vi "000 Driver Message.vi"(8 "error in":errorcluster caption="Error In", 11 "Queue In":T1={"UI"=refnum, "Message"=refnum, "Data"=refnum, "Caller"=refnum, "Name"="000 Common", "Data Path"=path "", "Class Path"=path "", "SubPanel"=refnum, "Project Name"="", "MNT"="", "Title"="", "Data Source"=refnum, "Queue List"={}, "VI"=refnum, "UE"=refnum}) -> (0 "error out":errorcluster caption="Error Out", 2 "Queue NUmber":i32, 3 "Queue Out":T1={"UI"=refnum, "Message"=refnum, "Data"=refnum, "Caller"=refnum, "Name"="000 Common", "Data Path"=path "", "Class Path"=path "", "SubPanel"=refnum, "Project Name"="", "MNT"="", "Title"="", "Data Source"=refnum, "Queue List"={}, "VI"=refnum, "UE"=refnum})   [LabVIEW 2020]
uses:
  000 Module Data Type.ctl
  Queue Message.ctl
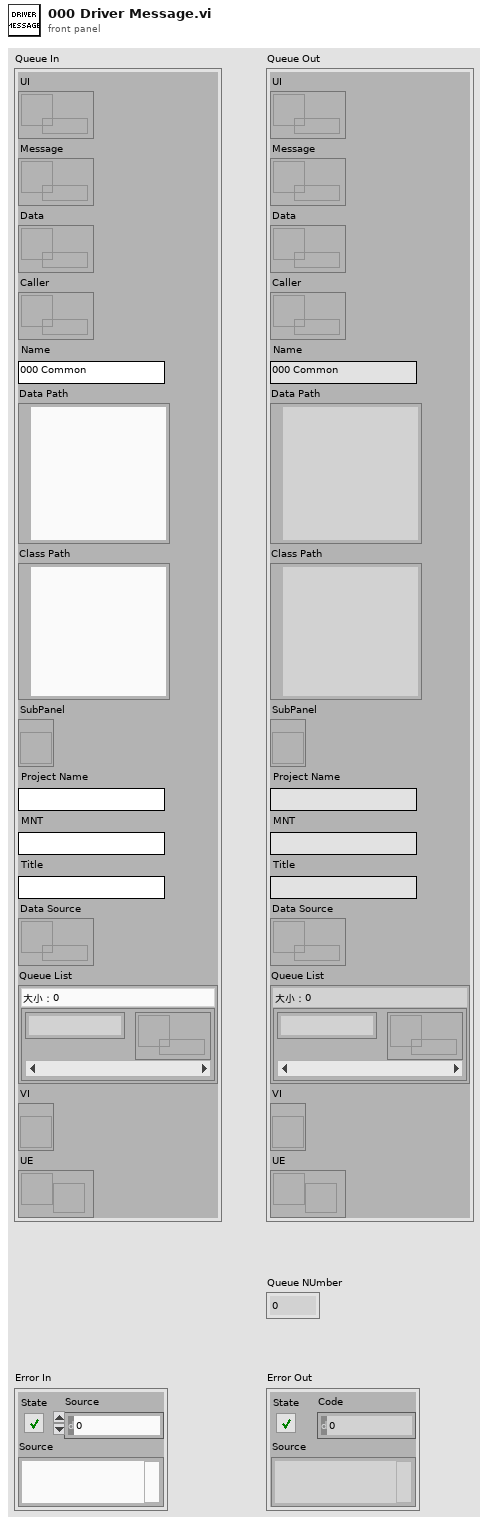
[diagram p1: front panel]
types:
  T1 = typedef "000 Module Data Type.ctl" = cluster{"UI":refnum<queue>, "Message":refnum<queue>, "Data":refnum<queue>, "Caller":refnum<queue>, "Name":string, "Data Path":path, "Class Path":path, "SubPanel":refnum<vi>, "Project Name":string, "MNT":string, "Title":string, "Data Source":refnum<queue>, "Queue List":map{string, refnum<queue>}, "VI":refnum<vi>, "UE":refnum<user-event>}
  T2 = enum32{"Invalid", "Standard", "Closed", "Hidden", "Minimized", "Maximized"}
  T3 = cluster{"Caller":refnum<queue>, "Message":refnum<queue>}
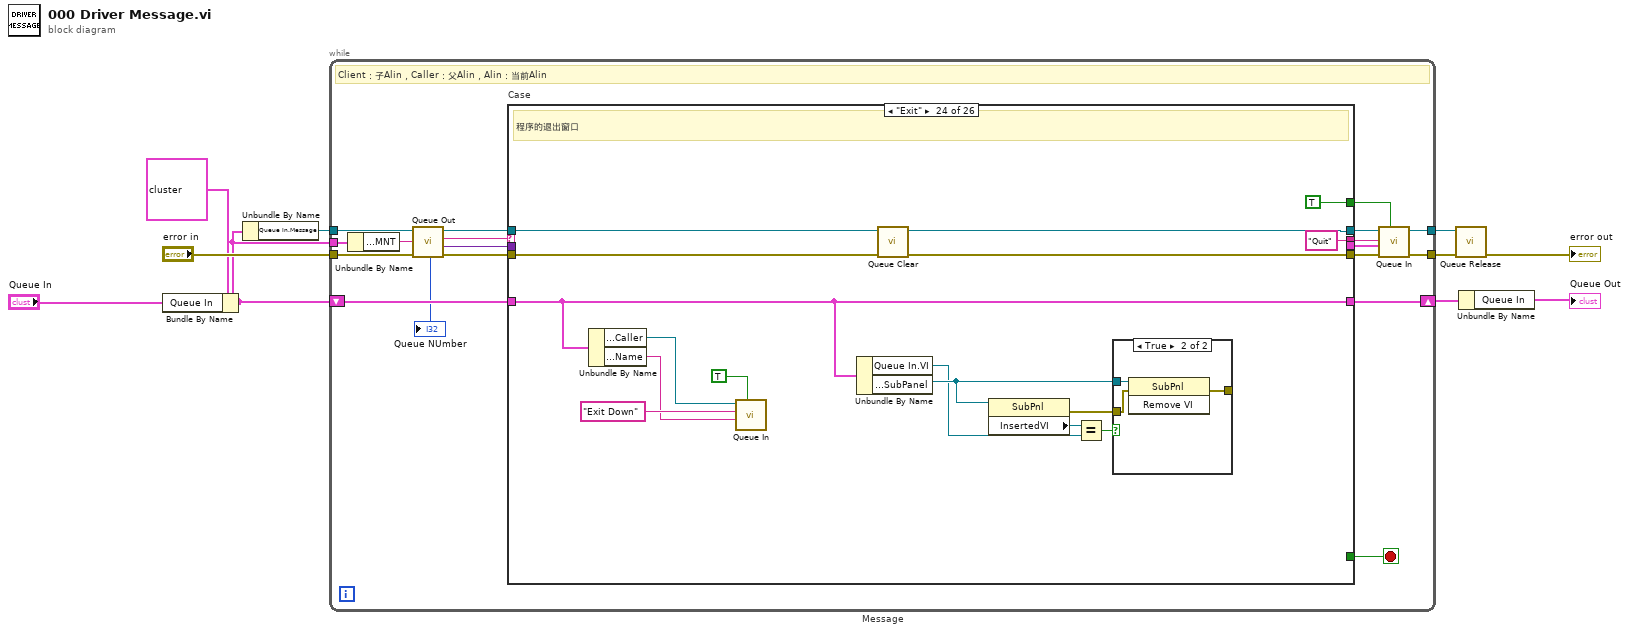
[diagram p0: block diagram]
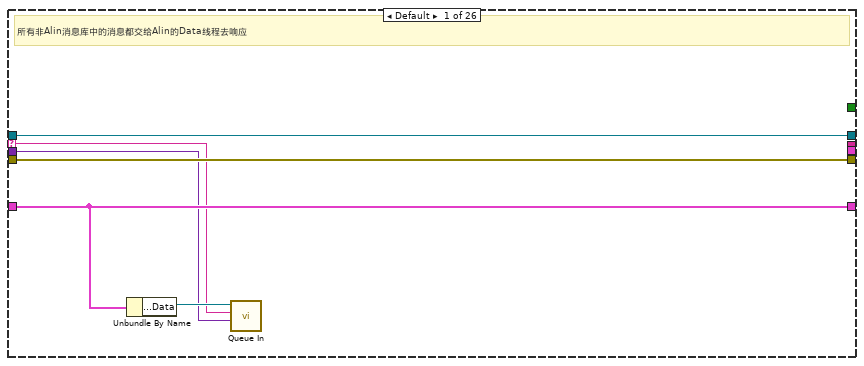
[diagram p2: hidden frame]
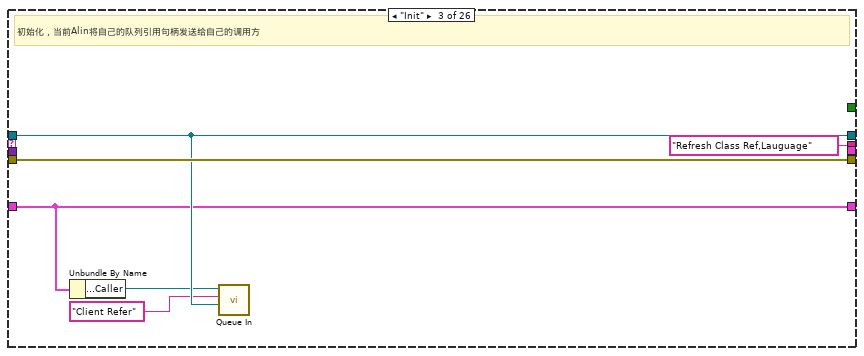
[diagram p4: hidden frame]
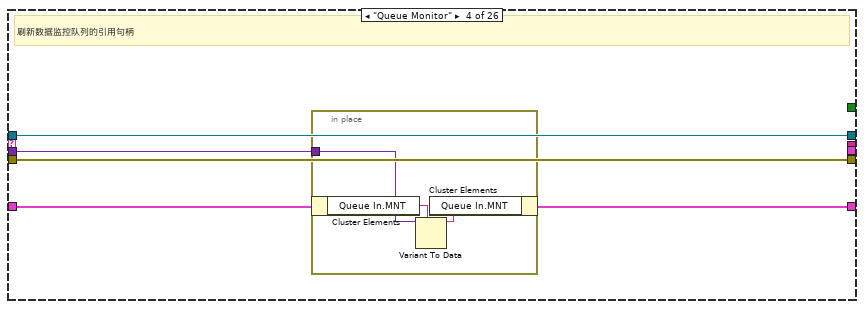
[diagram p5: hidden frame]
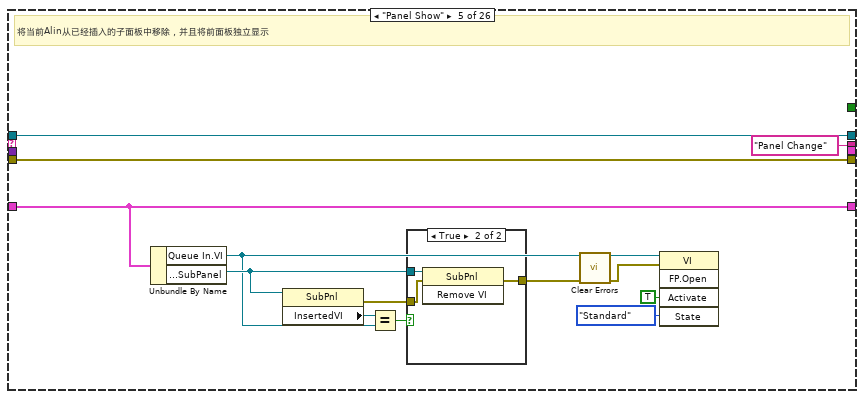
[diagram p6: hidden frame]
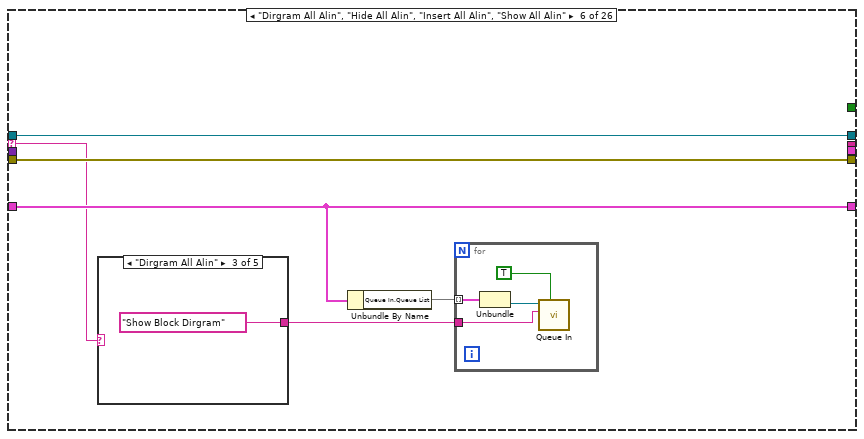
[diagram p8: hidden frame]
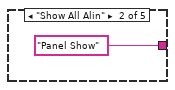
[diagram p10: hidden frame]
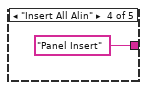
[diagram p11: hidden frame]
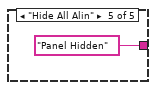
[diagram p12: hidden frame]
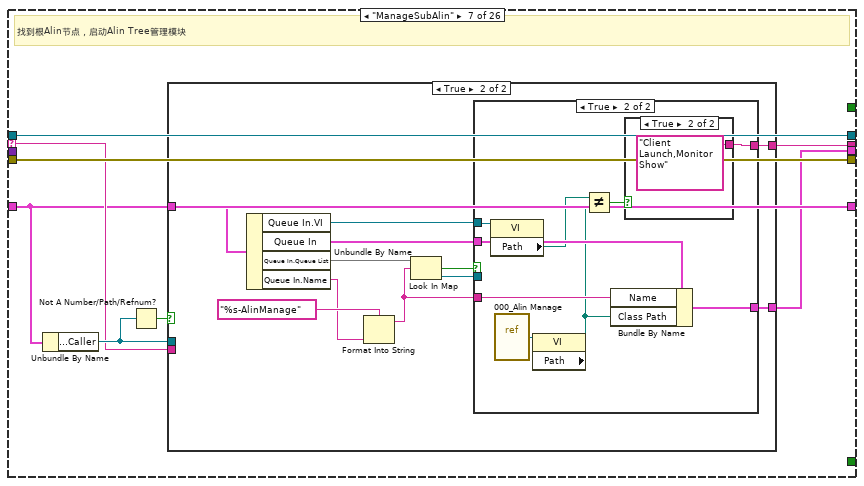
[diagram p13: hidden frame]
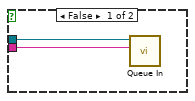
[diagram p14: hidden frame]
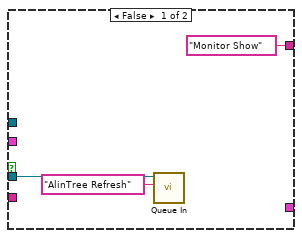
[diagram p15: hidden frame]
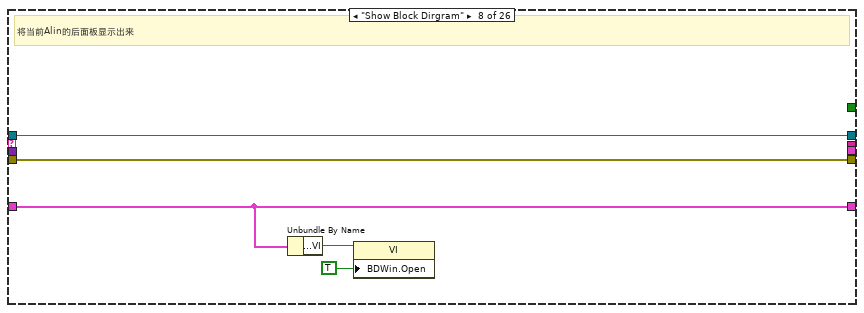
[diagram p17: hidden frame]
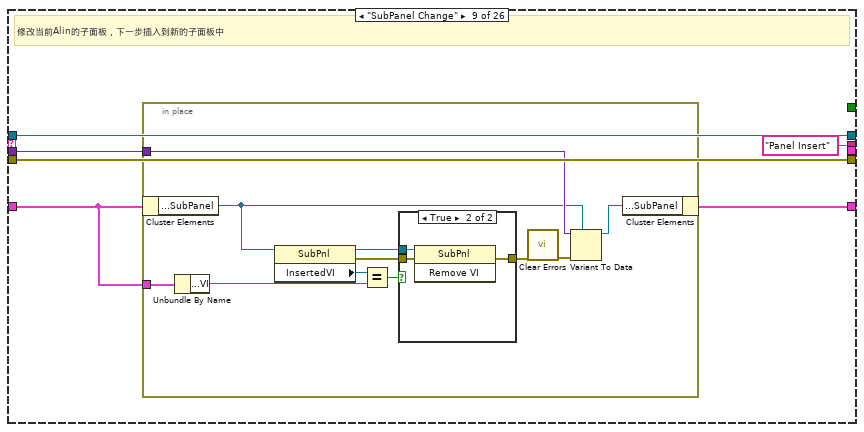
[diagram p18: hidden frame]
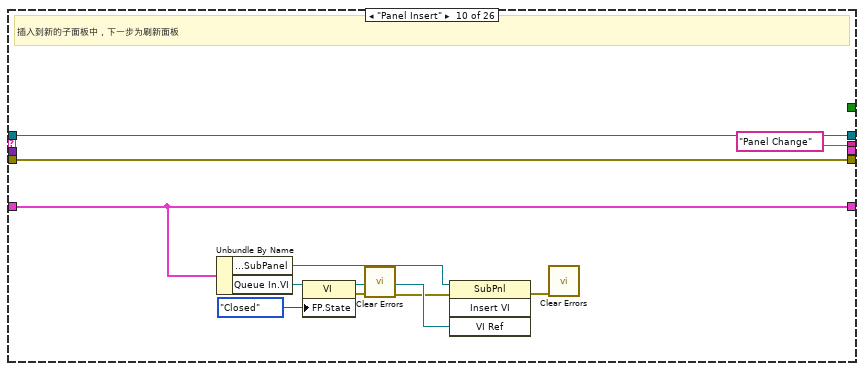
[diagram p20: hidden frame]
diagram:
  n1 = Bundle By Name ("按名称捆绑")(cluster=cluster{"Queue In":T1} {"Queue In"={"UI"=refnum, "Message"=refnum, "Data"=refnum, "Caller"=refnum, "Name"="000 Common", "Data Path"=path "", "Class Path"=path "", "SubPanel"=refnum, "Project Name"="", "MNT"="", "Title"="", "Data Source"=refnum, "Queue List"={}, "VI"=refnum, "UE"=refnum}}, "Queue In"="Queue In") -> (w3:cluster{"Queue In":T1})
  n2 = Unbundle By Name ("按名称解除捆绑")(w3) -> ("Queue In.Message"=w8:refnum<queue>)
  n3 = while "Message" {
    tunnel: w8 -> [w25]
    tunnel: [w22] -> w9
    tunnel: [w21] -> w10
    shift-right: [w18] -> w2
    shift-left: w3 -> [w17]
    tunnel: "error in" -> [w16]
    tunnel: w3 -> [w14]
    stop <- w29 stop-if-true
    # "Client：子Alin，Caller：父Alin，Alin：当前Alin"
    n4 = Unbundle By Name ("按名称解除捆绑")(w14) -> ("Queue In.MNT"=w13:string)
    n5 = call "Queue Out.vi"("error in (no error)"=w16, "Monitor"=w13, "Queue In"=w25) -> ("error out"=w28:errorcluster, "Data"=w26:variant, "Message"=w27:string, "Queue Out"=w24:refnum<queue>, "Queue NUmber"=→"Queue NUmber":i32)  [unwired: 4 in]
    n6 = case "Case" shown="\"Exit\"" w27 {
      selector: w27 -> [w31 _ _ _ _ w69 w86 _ _ _ _ w162 w173 _ _ w223 w235 w249 _ _ w278 _ _ _ _ _]
      tunnel: w24 -> [w35 w38 w43 w49 w65 w74 w90 w121 w127 w152 w158 w167 w176 w188 w205 w225 w237 w254 w265 w277 w287 w305 w324 w344 w351 w355]
      tunnel: w28 -> [w34 w37 w44 w48 w64 w73 w89 w120 w126 w151 w157 w166 w175 w191 w209 w224 w240 w253 w264 w276 w286 w304 w323 w342 w352 w354]
      tunnel: [w35 w38 w43 w49 w65 w74 w90 w121 w127 w152 w158 w167 w171 w188 w205 w225 w237 w254 w265 w277 w287 w305 w324 w343 w351 w355] -> w23
      tunnel: [w34 w37 w44 w48 w64 w73 w89 w120 w126 w151 w157 w166 w174 w191 w209 w224 w240 w253 w264 w276 w286 w304 w323 w341 w352 w354] -> w20
      tunnel: [_ _ "Refresh Class Ref,Lauguage" _ "Panel Change" _ w83 _ "Panel Insert" "Panel Change" _ _ _ "Send Client Refer" _ "Refresh Class Ref" "Refresh Class Ref" "" _ _ "Exit Check" w297 "Exit Check,Refresh Class Ref" "Quit" _ _] -> w19
      tunnel: [_ _ _ _ _ _ _ _ _ _ _ _ _ _ _ _ _ _ _ _ _ _ _ _ TRUE _] -> w29
      tunnel: w26 -> [w30 _ _ w45 _ _ _ _ w123 _ _ _ _ w189 w208 _ w236 _ _ w272 _ _ w320 _ _ _]
      tunnel: [w33 w36 w40 w46 w63 w72 w85 w119 w124 w150 w154 w165 w180 w190 w198 w222 w239 w248 w263 w275 w284 w303 w321 w330 w349 w353] -> w18
      tunnel: w17 -> [w33 w36 w40 w47 w63 w72 w85 w119 w122 w150 w154 w165 w180 w185 w198 w222 w239 w248 w263 w275 w284 w303 w322 w330 w349 w353]
      tunnel: [_ _ _ _ _ _ _ _ _ _ _ _ _ _ _ _ _ _ _ _ _ w296 _ TRUE _ _] -> w12
      tunnel: [_ _ _ _ _ _ w84 _ _ _ _ _ _ _ _ _ _ _ _ _ _ _ _ _ _ _] -> w11
      frame Default {
        # "所有非Alin消息库中的消息都交给Alin的Data线程去响应"
        n7 = Unbundle By Name(w33) -> ("Queue In.Data"=w32:refnum<queue>)
        n8 = call "Queue In.vi"("Data"=w30, "Message"=w31, "Queue In"=w32) -> ()  [unwired: 7 in, 2 out]
      }
      frame "====System Message Start===" {
      }
      frame "Init" {
        # "初始化，当前Alin将自己的队列引用句柄发送给自己的调用方"
        n9 = Unbundle By Name(w40) -> ("Queue In.Caller"=w41:refnum<queue>)
        n10 = call "Queue In.vi"("Data"=w43, "Message"="Client Refer", "Queue In"=w41) -> ()  [unwired: 7 in, 2 out]
      }
      frame "Queue Monitor" {
        # "刷新数据监控队列的引用句柄"
        n11 = in-place {
          in-place-border: w45 -> [w52]
          n12 = in-place-cluster #1(w47) -> ("Queue In.MNT"=w51:string)
          n13 = Variant To Data(type=w51, Variant=w52) -> (data=w50:string)  [unwired: 1 in, 1 out]
          n14 = in-place-cluster #1("Queue In.MNT"=w50) -> (w46:cluster{"Queue In":T1})
        }
      }
      frame "Panel Show" {
        # "将当前Alin从已经插入的子面板中移除，并且将前面板独立显示"
        n15 = Unbundle By Name(w63) -> ("Queue In.VI"=w55:refnum<vi>, "Queue In.SubPanel"=w57:refnum<vi>)
        n16 = property class="SubPnl"(reference=w57) -> (error out=w53:errorcluster, "InsertedVI"=w56:refnum<vi>)  [unwired: 1 in, 1 out]
        n17 = Equal?(x=w56, y=w55) -> (x = y?=w54:bool)
        n18 = case shown="True" w54 {
          tunnel: [_ w68] -> w62
          tunnel: w57 -> [_ w67]
          tunnel: w53 -> [_ w66]
          frame False {
          }
          frame True {
            n19 = invoke class="SubPnl" method="Remove VI"(reference=w67, error in=w66) -> (error out=w68:errorcluster)  [unwired: 1 in, 2 out]
          }
        }
        n20 = call <vilib>:"Clear Errors.vi"("error in (no error)"=w62) -> ("error out"=w59:errorcluster)  [unwired: 5 in, 1 out]
        n21 = invoke class="VI" method="FP.Open"(reference=w55, error in=w59, "Activate"=TRUE ("激活？"), "State"=T2."Standard" ("状态")) -> ()  [unwired: 1 in, 5 out]
      }
      frame "Dirgram All Alin", "Hide All Alin", "Insert All Alin", "Show All Alin" {
        n22 = case shown="\"Dirgram All Alin\"" w69 {
          tunnel: [_ "Panel Show" ("Message") "Show Block Dirgram" ("Message") "Panel Insert" ("Message") "Panel Hidden" ("Message")] -> w70
          frame Default {
          }
          frame "Show All Alin" {
          }
          frame "Dirgram All Alin" {
          }
          frame "Insert All Alin" {
          }
          frame "Hide All Alin" {
          }
        }
        n23 = Unbundle By Name(w72) -> ("Queue In.Queue List"=w71:map{string, refnum<queue>})
        n24 = for {
          tunnel: w71 -> [w82] mode=indexing
          tunnel: w70 -> [w80]
          n25 = Unbundle(w82) -> ("Client Refer"=w81:refnum<queue>)  [unwired: 1 out]
          n26 = call "Queue In.vi"("First"=TRUE, "Message"=w80, "Queue In"=w81) -> ()  [unwired: 7 in, 2 out]
        }
      }
      frame "ManageSubAlin" {
        # "找到根Alin节点，启动Alin Tree管理模块"
        n27 = Unbundle By Name(w85) -> ("Queue In.Caller"=w87:refnum<queue>)
        n28 = Not A Number/Path/Refnum?(number/path/refnum=w87) -> (NaN/Path/Refnum?=w88:bool)
        n29 = case shown="True" w88 {
          tunnel: w87 -> [w92 _]
          tunnel: w86 -> [w91 _]
          tunnel: w85 -> [_ w103]
          tunnel: [_ w96] -> w84
          tunnel: [_ w95] -> w83
          frame False {
            n30 = call "Queue In.vi"("Message"=w91, "Queue In"=w92) -> ()  [unwired: 8 in, 2 out]
          }
          frame True {
            n31 = Unbundle By Name(w103) -> ("Queue In.VI"=w93:refnum<vi>, "Queue In"=w102:T1, "Queue In.Queue List"=w101:map{string, refnum<queue>}, "Queue In.Name"=w99:string)
            n32 = Format Into String(format string="%s-AlinManage" ("格式字符串"), w99) -> (resulting string=w97:string)  [unwired: 2 in, 1 out]
            n33 = Look In Map(map=w101, key=w97) -> (key not found?=w98:bool, value=w94:refnum<queue>)  [unwired: 1 in]
            n34 = case shown="True" w98 {
              tunnel: w102 -> [_ w115]
              tunnel: w97 -> [_ w114]
              tunnel: [_ w112] -> w96
              tunnel: ["Monitor Show" w111] -> w95
              tunnel: w94 -> [w106 _]
              tunnel: w93 -> [_ w110]
              frame False {
                n35 = call "Queue In.vi"("Message"="AlinTree Refresh", "Queue In"=w106) -> ()  [unwired: 8 in, 2 out]
              }
              frame True {
                n36 = property class="VI"(reference=w110) -> ("Path"=w109:path)  [unwired: 1 in, 2 out]
                n37 = vi-ref "000_Alin Manage.vi"() -> (w113:refnum<vi>)
                n38 = property class="VI"(reference=w113) -> ("Path"=w108:path)  [unwired: 1 in, 2 out]
                n39 = Not Equal?(x=w109, y=w108) -> (x != y?=w107:bool)
                n40 = Bundle By Name(cluster=w115, "Name"=w114, "Class Path"=w108) -> (w112:T1)
                n41 = case shown="True" w107 {
                  tunnel: [_ "Client Launch,Monitor Show"] -> w111
                  frame False {
                  }
                  frame True {
                  }
                }
              }
            }
          }
        }
      }
      frame "Show Block Dirgram" {
        # "将当前Alin的后面板显示出来"
        n42 = Unbundle By Name(w119) -> ("Queue In.VI"=w117:refnum<vi>)
        n43 = property class="VI"(reference=w117, "BDWin.Open"=TRUE ("程序框图窗口:打开")) -> ()  [unwired: 1 in, 2 out]
      }
      frame "SubPanel Change" {
        # "修改当前Alin的子面板，下一步插入到新的子面板中"
        n44 = in-place {
          in-place-border: w123 -> [w138]
          in-place-border: w122 -> [w134]
          n45 = in-place-cluster #2(w122) -> ("Queue In.SubPanel"=w132:refnum<vi>)
          n46 = Unbundle By Name(w134) -> ("Queue In.VI"=w133:refnum<vi>)
          n47 = property class="SubPnl"(reference=w132) -> (reference out=w131:refnum<vi>, error out=w128:errorcluster, "InsertedVI"=w136:refnum<vi>)  [unwired: 1 in]
          n48 = Equal?(x=w136, y=w133) -> (x = y?=w135:bool)
          n49 = case shown="True" w135 {
            tunnel: [_ w141] -> w130
            tunnel: w131 -> [_ w140]
            tunnel: w128 -> [_ w139]
            frame False {
            }
            frame True {
              n50 = invoke class="SubPnl" method="Remove VI"(reference=w140, error in=w139) -> (error out=w141:errorcluster)  [unwired: 1 in, 2 out]
            }
          }
          n51 = call <vilib>:"Clear Errors.vi"("error in (no error)"=w130) -> ("error out"=w129:errorcluster)  [unwired: 5 in, 1 out]
          n52 = Variant To Data(error in=w129, type=w132, Variant=w138) -> (data=w137:refnum<vi>)  [unwired: 1 out]
          n53 = in-place-cluster #2("Queue In.SubPanel"=w137) -> (w124:cluster{"Queue In":T1})
        }
      }
      frame "Panel Insert" {
        # "插入到新的子面板中，下一步为刷新面板"
        n54 = Unbundle By Name(w150) -> ("Queue In.SubPanel"=w144:refnum<vi>, "Queue In.VI"=w147:refnum<vi>)
        n55 = property class="VI"(reference=w147, "FP.State"=T2."Closed" ("前面板窗口:状态")) -> (reference out=w145:refnum<vi>, error out=w146:errorcluster)  [unwired: 1 in]
        n56 = call <vilib>:"Clear Errors.vi"("error in (no error)"=w146) -> ("error out"=w143:errorcluster)  [unwired: 5 in, 1 out]
        n57 = invoke class="SubPnl" method="Insert VI"(reference=w144, error in=w143, "VI Ref"=w145) -> (error out=w142:errorcluster)  [unwired: 1 in, 3 out]
        n58 = call <vilib>:"Clear Errors.vi"("error in (no error)"=w142) -> ()  [unwired: 5 in, 2 out]
      }
      frame "Panel Hidden" {
        # "将当前Alin的前面板隐藏显示"
        n59 = Call Chain() -> (call chain=w156:string[])
        n60 = Unbundle By Name(w154) -> ("Queue In.VI"=w153:refnum<vi>)
        n61 = Array Size(array=w156) -> (size(s)=w155:i32)
        n62 = case shown="2.." w155 {
          tunnel: w156 -> [_ _]
          tunnel: w153 -> [_ w160]
          frame 0, Default {
          }
          frame 2.. {
            n63 = property class="VI"(reference=w160, "FP.State"=T2."Closed" ("前面板窗口:状态")) -> (error out=w159:errorcluster)  [unwired: 1 in, 1 out]
            n64 = call <vilib>:"Clear Errors.vi"("error in (no error)"=w159) -> ()  [unwired: 5 in, 2 out]
          }
        }
      }
      frame "Lauguage" {
        # "语言切换功能，详情查看语言切换模块，并且通知子Alin语言切换"
        n65 = Unbundle By Name(w165) -> ("Queue In.Queue List"=w163:map{string, refnum<queue>}, "Queue In.VI"=w164:refnum<vi>)
        n66 = call "LC Global Read VI Controls.vi"("vi reference"=w164) -> ()  [unwired: 10 in, 1 out]
        n67 = for {
          tunnel: w163 -> [w170] mode=indexing
          tunnel: w162 -> [w168]
          n68 = Unbundle(w170) -> ("Client Refer"=w169:refnum<queue>)  [unwired: 1 out]
          n69 = call "Queue In.vi"("Message"=w168, "Queue In"=w169) -> ()  [unwired: 8 in, 2 out]
        }
      }
      frame "Panel Change" {
        # "此分支可以由父Alin或者当前Alin触发，并且通知子Alin以及ALin面板刷新"
        n70 = Unbundle By Name(w180) -> ("Queue In.Queue List"=w179:map{string, refnum<queue>}, "Queue In.VI"=w178:refnum<vi>, "Queue In.UI"=w177:refnum<queue>)
        n71 = call "Queue In.vi"("Message"=w173, "Queue In"=w177) -> ()  [unwired: 8 in, 2 out]
        n72 = for {
          tunnel: w179 -> [w184] mode=indexing
          tunnel: w173 -> [w182]
          tunnel: w178 -> [w181]
          n73 = Unbundle By Name(w184) -> ("Client Refer"=w183:refnum<queue>)
          n74 = call "Queue In.vi"("Data"=w181, "Message"=w182, "Queue In"=w183) -> ()  [unwired: 7 in, 2 out]
        }
        n75 = call "Queue Clear.vi"("error in (no error)"=w175, "Delete?"=TRUE, "Filter"=w173, "Queue In"=w176) -> ("error out"=w174:errorcluster, "Queue Out"=w171:refnum<queue>)  [unwired: 6 in]
      }
      frame "Client Refer" {
        # "此分支是由子Alin发送至父Alin的，父Alin将子ALin的句柄存储到映射表中"
        n76 = Variant To Data(type=w188, Variant=w189) -> (data=w186:refnum<queue>)  [unwired: 1 in, 1 out]
        n77 = in-place {
          in-place-border: w186 -> [w195]
          n78 = in-place-cluster #3(w185) -> ("Queue In.Queue List"=w196:map{string, refnum<queue>})
          n79 = Get Queue Status(queue=w195) -> (queue out=w193:refnum<queue>, queue name=w194:string)  [unwired: 2 in, 6 out]
          n80 = Insert Into Map(map in=w196, key=w194, value=w193) -> (map out=w192:map{string, refnum<queue>})  [unwired: 2 out]
          n81 = in-place-cluster #3("Queue In.Queue List"=w192) -> (w190:cluster{"Queue In":T1})
        }
      }
      frame "Client Launch" {
        # "此分支是AlinFramewor的调用核心，所有Alin的执行状态必须为预先副本重入执行，并且遵循相同的输入句柄"
        n82 = Unbundle By Name(w198) -> ("Queue In"=w197:T1)
        n83 = Variant To Data(type=w197, Variant=w208) -> (data=w207:T1)  [unwired: 1 in, 1 out]
        n84 = Bundle By Name(cluster=w207, "Caller"=w205) -> (w206:T1)
        n85 = Unbundle By Name(w206) -> ("Class Path"=w204:path)
        n86 = Not A Number/Path/Refnum?(number/path/refnum=w204) -> (NaN/Path/Refnum?=w203:bool)
        n87 = Empty String/Path?(string/path=w204) -> (empty?=w202:bool)
        n88 = Not(x=w203) -> (.not. x?=w201:bool)
        n89 = Not(x=w202) -> (.not. x?=w200:bool)
        n90 = And(x=w201, y=w200) -> (x .and. y?=w199:bool)
        n91 = case shown="True" w199 {
          tunnel: w206 -> [_ w210]
          tunnel: w204 -> [_ w211]
          frame False {
          }
          frame True {
            n92 = Open VI Reference(type specifier VI Refnum (for type only)=refnum<vi> refnum ("类型说明符VI引用句柄（仅用于类型）"), vi path=w211, options=192 ("选项")) -> (vi reference=w215:refnum<vi>)  [unwired: 3 in, 1 out]
            n93 = call-by-ref "开始异步调用"(reference=w215, "Queue Ref In"=w210) -> (reference out=w212:refnum<vi>, error out=w213:errorcluster)  [unwired: 12 in]
            n94 = Close Reference(reference=w212, error in (no error)=w213) -> ()  [unwired: 1 out]
          }
        }
      }
      frame "Send Client Refer" {
        # "此分支已经被抛弃使用，可以忽略"
        n95 = Unbundle By Name(w222) -> ("Queue In.Data"=w219:refnum<queue>, "Queue In.UI"=w220:refnum<queue>, "Queue In.Queue List"=w221:map{string, refnum<queue>})
        n96 = Build Array(w219, w220) -> (w218:refnum<queue>[])
        n97 = for {
          tunnel: w223 -> [w228]
          tunnel: w221 -> [w227]
          tunnel: w218 -> [w226] mode=indexing
          n98 = call "Queue In.vi"("Data"=w227, "Message"=w228, "Queue In"=w226) -> ()  [unwired: 7 in, 2 out]
        }
      }
      frame "Send Client&Self" {
        # "将Alin句柄以及Caller的句柄发送给模块管理工具"
        n99 = Unbundle By Name(w239) -> ("Queue In.Caller"=w229:refnum<queue>, "Queue In.Message"=w232:refnum<queue>, "Queue In.Queue List"=w231:map{string, refnum<queue>})
        n100 = Variant To Data(type=w237, Variant=w236) -> (data=w234:refnum<queue>)  [unwired: 1 in, 1 out]
        n101 = Bundle("Caller"=w229, "Message"=w232) -> (w230:T3)  [unwired: 1 in]
        n102 = call "Queue In.vi"("Data"=w230, "Message"="Receive Client&Self", "Queue In"=w234) -> ()  [unwired: 7 in, 2 out]
        n103 = for {
          tunnel: w231 -> [w244] mode=indexing
          tunnel: w236 -> [w243]
          tunnel: w235 -> [w242]
          n104 = Unbundle(w244) -> ("Client Refer"=w245:refnum<queue>)  [unwired: 1 out]
          n105 = call "Queue In.vi"("First"=TRUE, "Data"=w243, "Message"=w242, "Queue In"=w245) -> ()  [unwired: 6 in, 2 out]
        }
      }
      frame "Refresh Class Ref" {
        # "如果子Alin注册到程序中会在子Alin的Init分支将句柄发送至父Alin的Send Client Refer分支，发送完成后将句柄更新到Alin的Dara以及UI线程"
        n106 = Unbundle By Name(w248) -> ("Queue In.Data"=w251:refnum<queue>, "Queue In.UI"=w252:refnum<queue>, "Queue In"=w246:T1)
        n107 = Build Array(w251, w252) -> (w250:refnum<queue>[])
        n108 = for {
          tunnel: w246 -> [w258]
          tunnel: w250 -> [w257] mode=indexing
          tunnel: w249 -> [w256]
          n109 = call "Queue In.vi"("Data"=w258, "Message"=w256, "Queue In"=w257) -> ("error out"=w255:errorcluster)  [unwired: 7 in, 1 out]
          n110 = call <vilib>:"Clear Errors.vi"("error in (no error)"=w255) -> ()  [unwired: 5 in, 2 out]
        }
      }
      frame "Open Data Path" {
        # "打开配置目录"
        n111 = Unbundle By Name(w263) -> ("Queue In.Data Path"=w262:path)
        n112 = call <vilib>:"Check if File or Folder Exists.vi"("path"=w262) -> ("error out"=w259:errorcluster, "file or folder exists?"=w261:bool, "dup path"=w260:path)  [unwired: 8 in]
        n113 = case shown="True" w261 {
          tunnel: w260 -> [_ w267]
          tunnel: w259 -> [_ w266]
          frame False {
          }
          frame True {
            n114 = Empty String/Path?(string/path=w267) -> (empty?=w268:bool)
            n115 = case shown="False" w268 {
              tunnel: w267 -> [w271 _]
              tunnel: w266 -> [w270 _]
              frame False {
                n116 = call <vilib>:"Show in File System.vi"("error in (no error)"=w270, "file or directory path"=w271) -> ("error out"=w269:errorcluster)  [unwired: 9 in]
                n117 = call <vilib>:"Clear Errors.vi"("error in (no error)"=w269) -> ()  [unwired: 5 in, 2 out]
              }
              frame True {
              }
            }
          }
        }
      }
      frame "Error" {
        # "错误处理线程"
        n118 = Unbundle By Name(w275) -> ("Queue In.Data Path"=w274:path, "Queue In.Name"=w273:string)
        n119 = call "000 Write Error.vi"("Data"=w272, "Name"=w273, "Path"=w274) -> ()  [unwired: 7 in, 2 out]
      }
      frame "Exit Prepare" {
        # "此分支可以由Alin的UI或者父Alin发送，退出前准备，并通知所有的子Alin现在准备退出了"
        n120 = Unbundle By Name(w284) -> ("Queue In.UI"=w281:refnum<queue>, "Queue In.Data"=w280:refnum<queue>, "Queue In.Queue List"=w285:map{string, refnum<queue>})
        n121 = Build Array(w281, w280) -> (w279:refnum<queue>[])
        n122 = for {
          tunnel: w279 -> [w290] mode=indexing
          tunnel: w278 -> [w289]
          n123 = call "Queue In.vi"("First"=TRUE, "Message"=w289, "Queue In"=w290) -> ()  [unwired: 7 in, 2 out]
        }
        n124 = for {
          tunnel: w285 -> [w295] mode=indexing
          tunnel: w278 -> [w293]
          tunnel: [w291] -> w282
          n125 = Unbundle By Name(w295) -> ("Client Refer"=w294:refnum<queue>)
          n126 = call "Queue In.vi"("First"=TRUE, "Message"=w293, "Queue In"=w294) -> ("error out"=w291:errorcluster)  [unwired: 7 in, 1 out]
        }
        n127 = call <vilib>:"Clear Errors.vi"("error in (no error)"=w282) -> ()  [unwired: 5 in, 2 out]
      }
      frame "Exit Check" {
        # "子Alin退出后，会将自己退出的消息在子Alin的Exit分支发送至父Alin的Exit Down分支，父Alin接收到后会将子ALin的句柄从映射表中删除，并且检查此分支，若所有的子Alin全部退出了的话就释放自己"
        n128 = Unbundle By Name(w303) -> ("Queue In.UE"=w298:refnum<user-event>, "Queue In.UI"=w299:refnum<queue>, "Queue In.Data"=w300:refnum<queue>, "Queue In.Queue List"=w302:map{string, refnum<queue>})
        n129 = Empty Collection?(1:w302) -> (0:w301:bool)
        n130 = case shown="True" w301 {
          tunnel: w300 -> [_ w312]
          tunnel: w299 -> [_ w311]
          tunnel: w298 -> [_ w310]
          tunnel: [_ w308] -> w297
          tunnel: [_ TRUE] -> w296
          frame False {
          }
          frame True {
            w308 = "Exit" ("事件数据")
            n131 = Build Array(w311, w312) -> (w313:refnum<queue>[])
            n132 = Not A Number/Path/Refnum?(number/path/refnum=w310) -> (NaN/Path/Refnum?=w309:bool)
            n133 = for {
              tunnel: w313 -> [w318] mode=indexing
              tunnel: w308 -> [w317]
              tunnel: TRUE ("First") -> [w316]
              n134 = call "Queue In.vi"("First"=w316, "Message"=w317, "Queue In"=w318) -> ()  [unwired: 7 in, 2 out]
            }
            n135 = case shown="False" w309 {
              tunnel: w308 -> [w315 _]
              tunnel: w310 -> [w314 _]
              frame False {
                n136 = Generate User Event(user event=w314, event data cluster=w315) -> ()  [unwired: 2 in, 2 out]
              }
              frame True {
              }
            }
          }
        }
      }
      frame "Exit Down" {
        # "此分支是由子Alin发送至父Alin的，父Alin接收到后会将子ALin的句柄从映射表中删除"
        n137 = in-place {
          in-place-border: w320 -> [w329]
          n138 = in-place-cluster #4(w322) -> ("Queue In.Queue List"=w327:map{string, refnum<queue>})
          n139 = Variant To Data(type="", Variant=w329) -> (data=w326:string)  [unwired: 1 in, 1 out]
          n140 = Remove From Map(10:w326, 11:w327) -> (3:w325:map{string, refnum<queue>})  [unwired: 2 out]
          n141 = in-place-cluster #4("Queue In.Queue List"=w325) -> (w321:cluster{"Queue In":T1})
        }
      }
      frame "Exit" {
        # "程序的退出窗口"
        n142 = Unbundle By Name(w330) -> ("Queue In.Caller"=w339:refnum<queue>, "Queue In.Name"=w338:string)
        n143 = call "Queue In.vi"("First"=TRUE, "Data"=w338, "Message"="Exit Down", "Queue In"=w339) -> ()  [unwired: 6 in, 2 out]
        n144 = Unbundle By Name(w330) -> ("Queue In.VI"=w333:refnum<vi>, "Queue In.SubPanel"=w335:refnum<vi>)
        n145 = call "Queue Clear.vi"("error in (no error)"=w342, "Queue In"=w344) -> ("error out"=w341:errorcluster, "Queue Out"=w343:refnum<queue>)  [unwired: 8 in]
        n146 = property class="SubPnl"(reference=w335) -> (error out=w331:errorcluster, "InsertedVI"=w334:refnum<vi>)  [unwired: 1 in, 1 out]
        n147 = Equal?(x=w334, y=w333) -> (x = y?=w332:bool)
        n148 = case shown="True" w332 {
          tunnel: [_ w348] -> _
          tunnel: w335 -> [_ w347]
          tunnel: w331 -> [_ w346]
          frame False {
          }
          frame True {
            n149 = invoke class="SubPnl" method="Remove VI"(reference=w347, error in=w346) -> (error out=w348:errorcluster)  [unwired: 1 in, 2 out]
          }
        }
      }
      frame "Quit" {
        # "退出While循环，并且释放队列引用句柄"
      }
      frame "====System Message Stopt===" {
      }
    }
    n150 = call "Queue In.vi"("First"=w12, "error in (no error)"=w20, "Data"=w11, "Message"=w19, "Queue In"=w23) -> ("error out"=w21:errorcluster, "Queue Out"=w22:refnum<queue>)  [unwired: 5 in]
  }
  n151 = call "Queue Release.vi"("error in (no error)"=w10, "Queue In"=w9) -> ("error out"=→"error out":errorcluster)  [unwired: 9 in]
  n152 = Unbundle By Name ("按名称解除捆绑")(w2) -> ("Queue In"=→"Queue Out":T1)
